vi "Simula stato PLC_1.vi"(11 "USCITE PLC":T1) -> (3 "STATO PLC":T4)   [LabVIEW 2019]
uses:
  STATO PLC 1.ctl
  Uscite PLC 1.ctl
  controls/statoAO_plc_1.ctl
  StatoDO_PLC_1.ctl
panel:
  in  "AI plc.Allarmi 1":dbl format="%#_13g"
  in  "Stato DI_PLC.Sistema OK":bool=TRUE
  in  "Stato DI_PLC.Rotore bloccato":bool
  in  "Stato DI_PLC.Reset da pulsantiera":bool
  in  "Stato DI_PLC.Stop da pulsantiera":bool
  in  "Stato DI_PLC.Start da pulsantiera":bool
  # "StatoDO_PLC.ctlUSCITE PLC : TYPE DEF"
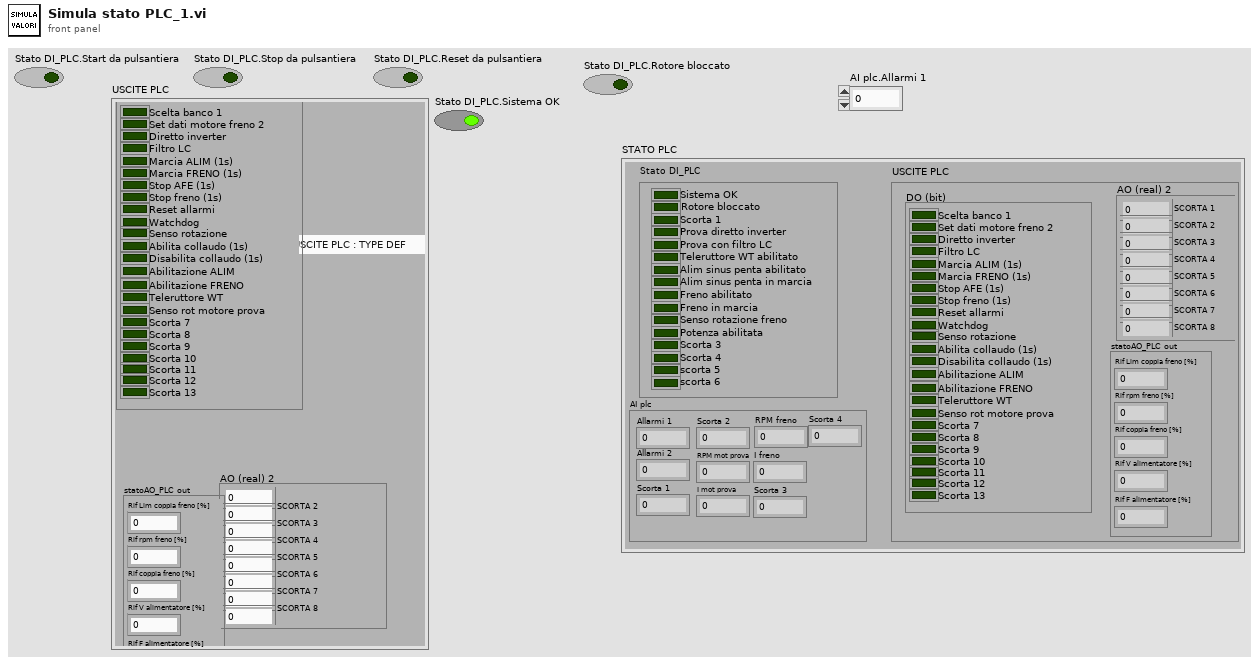
[diagram p1: front panel]
types:
  T1 = typedef "Uscite PLC 1.ctl" = cluster{"AO (real) 2":cluster{"SCORTA 1":dbl, "SCORTA 2":dbl, "SCORTA 3":dbl, "SCORTA 4":dbl, "SCORTA 5":dbl, "SCORTA 6":dbl, "SCORTA 7":dbl, "SCORTA 8":dbl}, "statoAO_PLC out":T2, "DO (bit)":T3}
  T2 = typedef "statoAO_plc_1.ctl" = cluster{"Rif Lim coppia freno [%]":dbl, "Rif rpm freno [%]":dbl, "Rif coppia freno [%]":dbl, "Rif V alimentatore [%]":dbl, "Rif F alimentatore [%]":dbl}
  T3 = typedef "StatoDO_PLC_1.ctl" = cluster{"Scelta banco 1":bool, "Set dati motore freno 2":bool, "Diretto inverter":bool, "Filtro LC":bool, "Marcia ALIM (1s)":bool, "Marcia FRENO (1s)":bool, "Stop AFE (1s)":bool, "Stop freno (1s)":bool, "Reset allarmi":bool, "Watchdog":bool, "Senso rotazione":bool, "Abilita collaudo (1s)":bool, "Disabilita collaudo (1s)":bool, "Abilitazione ALIM":bool, "Abilitazione FRENO":bool, "Teleruttore WT":bool, "Senso rot motore prova":bool, "Scorta 7":bool, "Scorta 8":bool, "Scorta 9":bool, "Scorta 10":bool, "Scorta 11":bool, "Scorta 12":bool, "Scorta 13":bool}
  T4 = typedef "STATO PLC 1.ctl" = cluster{"USCITE PLC":T1, "Stato DI_PLC":cluster{"Sistema OK":bool, "Rotore bloccato":bool, "Scorta 1":bool, "Prova diretto inverter":bool, "Prova con filtro LC":bool, "Teleruttore WT abilitato":bool, "Alim sinus penta abilitato":bool, "Alim sinus penta in marcia":bool, "Freno abilitato":bool, "Freno in marcia":bool, "Senso rotazione freno":bool, "Potenza abilitata":bool, "Scorta 3":bool, "Scorta 4":bool, "scorta 5":bool, "scorta 6":bool}, "AI plc":cluster{"Allarmi 1":dbl, "Allarmi 2":dbl, "Scorta 1":dbl, "Scorta 2":dbl, "RPM mot prova":dbl, "I mot prova":dbl, "RPM freno":dbl, "I freno":dbl, "Scorta 3":dbl, "Scorta 4":dbl}}
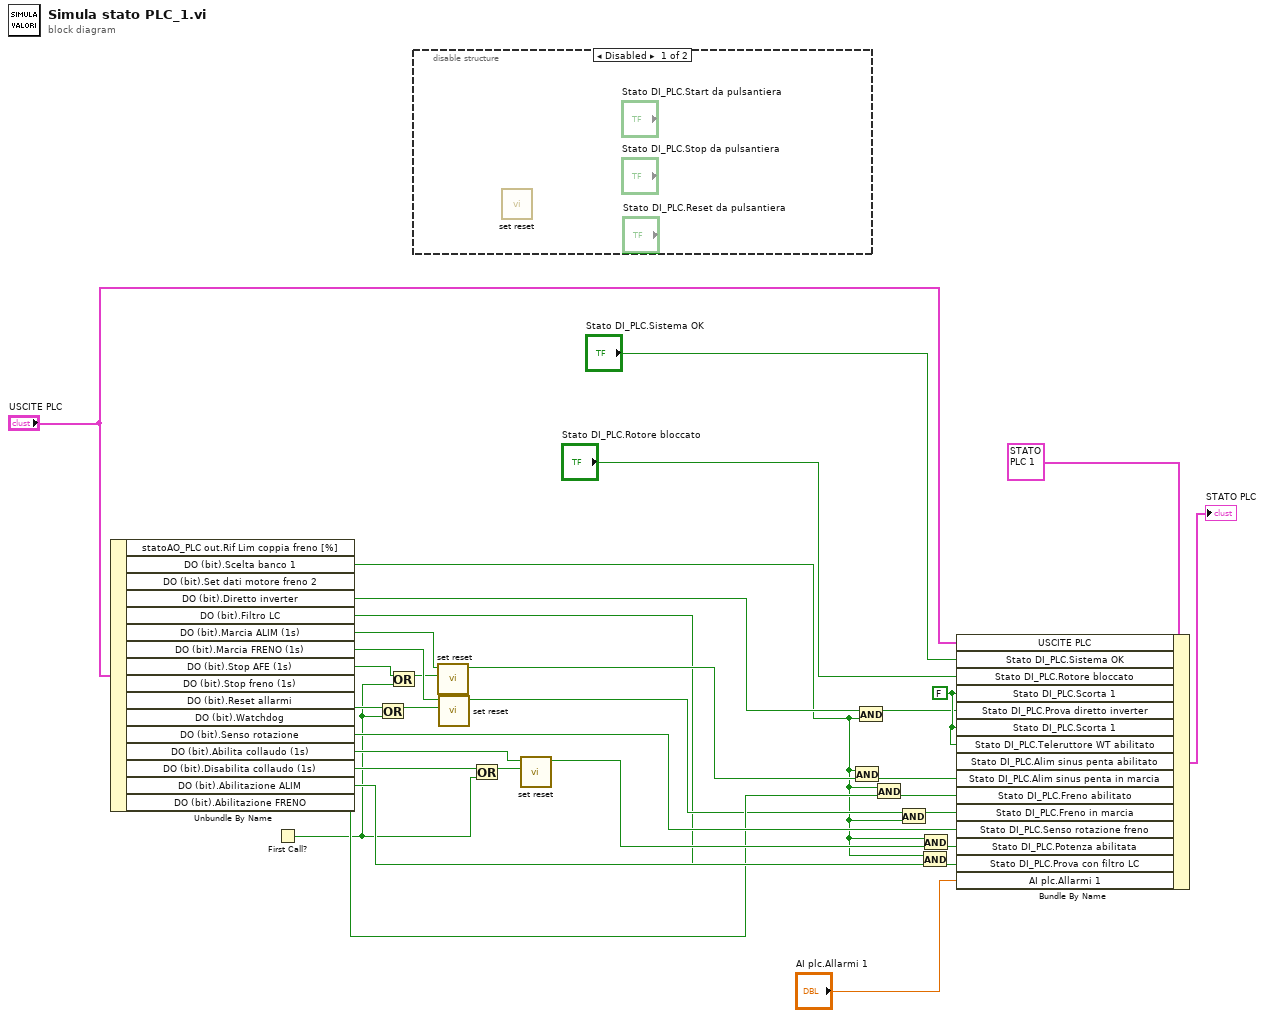
[diagram p0: block diagram]
diagram:
  w9 = FALSE ("Stato DI_PLC.Misura resistomat abilitata")
  n1 = Unbundle By Name("USCITE PLC") -> ("DO (bit).Scelta banco 1"=w2:bool, "DO (bit).Diretto inverter"=w11:bool, "DO (bit).Filtro LC"=w10:bool, "DO (bit).Marcia ALIM (1s)"=w20:bool, "DO (bit).Marcia FRENO (1s)"=w19:bool, "DO (bit).Stop AFE (1s)"=w18:bool, "DO (bit).Stop freno (1s)"=w17:bool, "DO (bit).Senso rotazione"=w25:bool, "DO (bit).Abilita collaudo (1s)"=w28:bool, "DO (bit).Disabilita collaudo (1s)"=w27:bool, "DO (bit).Abilitazione ALIM"=w22:bool, "DO (bit).Abilitazione FRENO"=w21:bool)  [unwired: 4 out]
  n2 = First Call?() -> (First Call?: T/F=w14:bool)
  n3 = Or(x=w17, y=w14) -> (x .or. y?=w15:bool)
  n4 = Or(x=w18, y=w14) -> (x .or. y?=w16:bool)
  n5 = disable-structure shown="Disabled" {
    frame Disabled {
      n6 = call "set reset.vi"() -> ()  [unwired: 11 in, 1 out]
    }
    frame Enabled {
    }
  }
  n7 = call "set reset.vi"("reset"=w16, "set"=w20) -> ("Boolean"=w13:bool)  [unwired: 9 in]
  n8 = call "set reset.vi"("reset"=w15, "set"=w19) -> ("Boolean"=w12:bool)  [unwired: 9 in]
  n9 = Or(x=w27, y=w14) -> (x .or. y?=w23:bool)
  n10 = call "set reset.vi"("reset"=w23, "set"=w28) -> ("Boolean"=w24:bool)  [unwired: 9 in]
  n11 = And(x=w2, y=w13) -> (x .and. y?=w4:bool)
  n12 = And(x=w11, y=w2) -> (x .and. y?=w3:bool)
  n13 = And(x=w2, y=w21) -> (x .and. y?=w5:bool)
  n14 = And(x=w12, y=w2) -> (x .and. y?=w6:bool)
  n15 = And(x=w2, y=w10) -> (x .and. y?=w7:bool)
  n16 = And(x=w2, y=w24) -> (x .and. y?=w8:bool)
  n17 = Bundle By Name(cluster=T4 {"USCITE PLC"={"AO (real) 2"={"SCORTA 1"=0.0, "SCORTA 2"=0.0, "SCORTA 3"=0.0, "SCORTA 4"=0.0, "SCORTA 5"=0.0, "SCORTA 6"=0.0, "SCORTA 7"=0.0, "SCORTA 8"=0.0}, "statoAO_PLC out"={"Rif Lim coppia freno [%]"=0.0, "Rif rpm freno [%]"=0.0, "Rif coppia freno [%]"=0.0, "Rif V alimentatore [%]"=0.0, "Rif F alimentatore [%]"=0.0}, "DO (bit)"={"Scelta banco 1"=FALSE, "Set dati motore freno 2"=FALSE, "Diretto inverter"=FALSE, "Filtro LC"=FALSE, "Marcia ALIM (1s)"=FALSE, "Marcia FRENO (1s)"=FALSE, "Stop AFE (1s)"=FALSE, "Stop freno (1s)"=FALSE, "Reset allarmi"=FALSE, "Watchdog"=FALSE, "Senso rotazione"=FALSE, "Abilita collaudo (1s)"=FALSE, "Disabilita collaudo (1s)"=FALSE, "Abilitazione ALIM"=FALSE, "Abilitazione FRENO"=FALSE, "Teleruttore WT"=FALSE, "Senso rot motore prova"=FALSE, "Scorta 7"=FALSE, "Scorta 8"=FALSE, "Scorta 9"=FALSE, "Scorta 10"=FALSE, "Scorta 11"=FALSE, "Scorta 12"=FALSE, "Scorta 13"=FALSE}}, "Stato DI_PLC"={"Sistema OK"=FALSE, "Rotore bloccato"=FALSE, "Scorta 1"=FALSE, "Prova diretto inverter"=FALSE, "Prova con filtro LC"=FALSE, "Teleruttore WT abilitato"=FALSE, "Alim sinus penta abilitato"=FALSE, "Alim sinus penta in marcia"=FALSE, "Freno abilitato"=FALSE, "Freno in marcia"=FALSE, "Senso rotazione freno"=FALSE, "Potenza abilitata"=FALSE, "Scorta 3"=FALSE, "Scorta 4"=FALSE, "scorta 5"=FALSE, "scorta 6"=FALSE}, "AI plc"={"Allarmi 1"=0.0, "Allarmi 2"=0.0, "Scorta 1"=0.0, "Scorta 2"=0.0, "RPM mot prova"=0.0, "I mot prova"=0.0, "RPM freno"=0.0, "I freno"=0.0, "Scorta 3"=0.0, "Scorta 4"=0.0}} ("STATO PLC"), "USCITE PLC"="USCITE PLC", "Stato DI_PLC.Sistema OK"="Stato DI_PLC.Sistema OK", "Stato DI_PLC.Rotore bloccato"="Stato DI_PLC.Rotore bloccato", "Stato DI_PLC.Scorta 1"=w9, "Stato DI_PLC.Prova diretto inverter"=w3, "Stato DI_PLC.Scorta 1"=w9, "Stato DI_PLC.Teleruttore WT abilitato"=w9, "Stato DI_PLC.Alim sinus penta abilitato"=w22, "Stato DI_PLC.Alim sinus penta in marcia"=w4, "Stato DI_PLC.Freno abilitato"=w5, "Stato DI_PLC.Freno in marcia"=w6, "Stato DI_PLC.Senso rotazione freno"=w25, "Stato DI_PLC.Potenza abilitata"=w8, "Stato DI_PLC.Prova con filtro LC"=w7, "AI plc.Allarmi 1"="AI plc.Allarmi 1") -> (→"STATO PLC":T4)
